vi "Run Child.vi"(8 "error in (no error)":errorcluster, 9 "Working Path":path, 10 "UI":refnum<class "UI.lvclass">, 11 "Install in":refnum<class "Install.lvclass">) -> (0 "error out":errorcluster, 3 "Install out":refnum<class "Install.lvclass">)   [LabVIEW 2020, in "Install.lvlib" / "Install.lvclass"]
uses:
  Install.lvclass
  build/ppl/neg-pkg.lvlibp/neg-pkg/UI/UI.lvclass
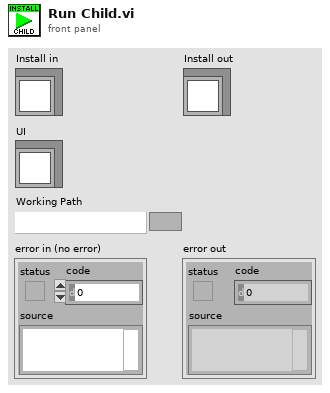
[diagram p1: front panel]
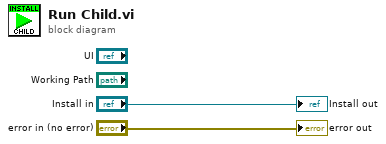
[diagram p0: block diagram]
diagram:
  "error out" <- "error in (no error)"
  "Install out" <- "Install in"
